vi "PenaltyAttackerSkill.vi"(8 "error in (no error)":errorcluster, 9 "Game":refnum<class "Game.lvclass">, 10 "Robot":refnum<class "Robot.lvclass">, 11 "PenaltyAttackerSkill in":refnum<class "PenaltyAttackerSkill.lvclass">) -> (0 "error out":errorcluster, 2 "Robot out":refnum<class "Robot.lvclass">, 3 "PenaltyAttackerSkill out":refnum<class "PenaltyAttackerSkill.lvclass">)   [LabVIEW 2018, in "PenaltyAttackerSkill.lvclass"]
uses:
  PenaltyAttackerSkill.lvclass
  Robot_class/Robot.lvclass
  C:/Users/yugon/Desktop/SSL_AI/SSL_AI/Object_class/Object.lvclass
  Game_class/Game.lvclass
  Utilities_class/Utilities.lvclass
  Game_class/Game.lvclass/Game.ctl
  Parameters_class/Parameters.lvclass/Parameters.ctl
  Team_class/Team.lvclass/Team.ctl
  Referee_class/Referee.lvclass/Referee.ctl
  Object_class/Object.lvclass/Object.ctl
  Robot_class/Robot.lvclass/Robot.ctl
  Team_class/Read RobotRef.vi
  Game_class/Read Parameters.lvclass.vi
  Parameters_class/Read KickForce.vi
  Object_class/Read x.vi
  Object_class/Read y.vi
  Game_class/Read FieldRef.vi
  Game_class/Read BallRef.vi
  Game_class/Read Referee.vi
  Game_class/Read AllyRef.vi
  Game_class/Read EnemyRef.vi
  Parameters_class/Read AttakingOurselves.vi
  Referee_class/Read enemy_goalie_id.vi
  Referee_class/Read our_goalie_id.vi
  Robot_class/Write dest_orientation.vi
  Robot_class/Write dest_x.vi
  Robot_class/Write dest_y.vi
  Robot_class/Write kick_x.vi
  Enemy_class/Enemy.lvclass
  C:/Users/yugon/Desktop/SSL_AI/SSL_AI/Team_class/Team.lvclass
  Ally_class/Ally.lvclass
  Ball_class/Ball.lvclass
  Referee_class/Referee.lvclass
  Parameters_class/Parameters.lvclass
  Field_class/Field.lvclass
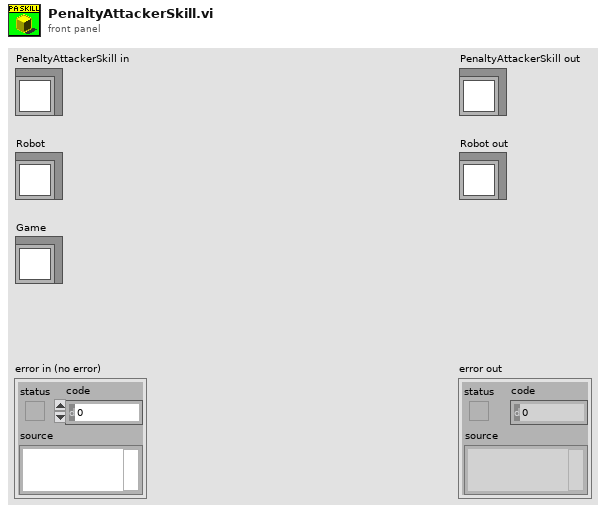
[diagram p1: front panel]
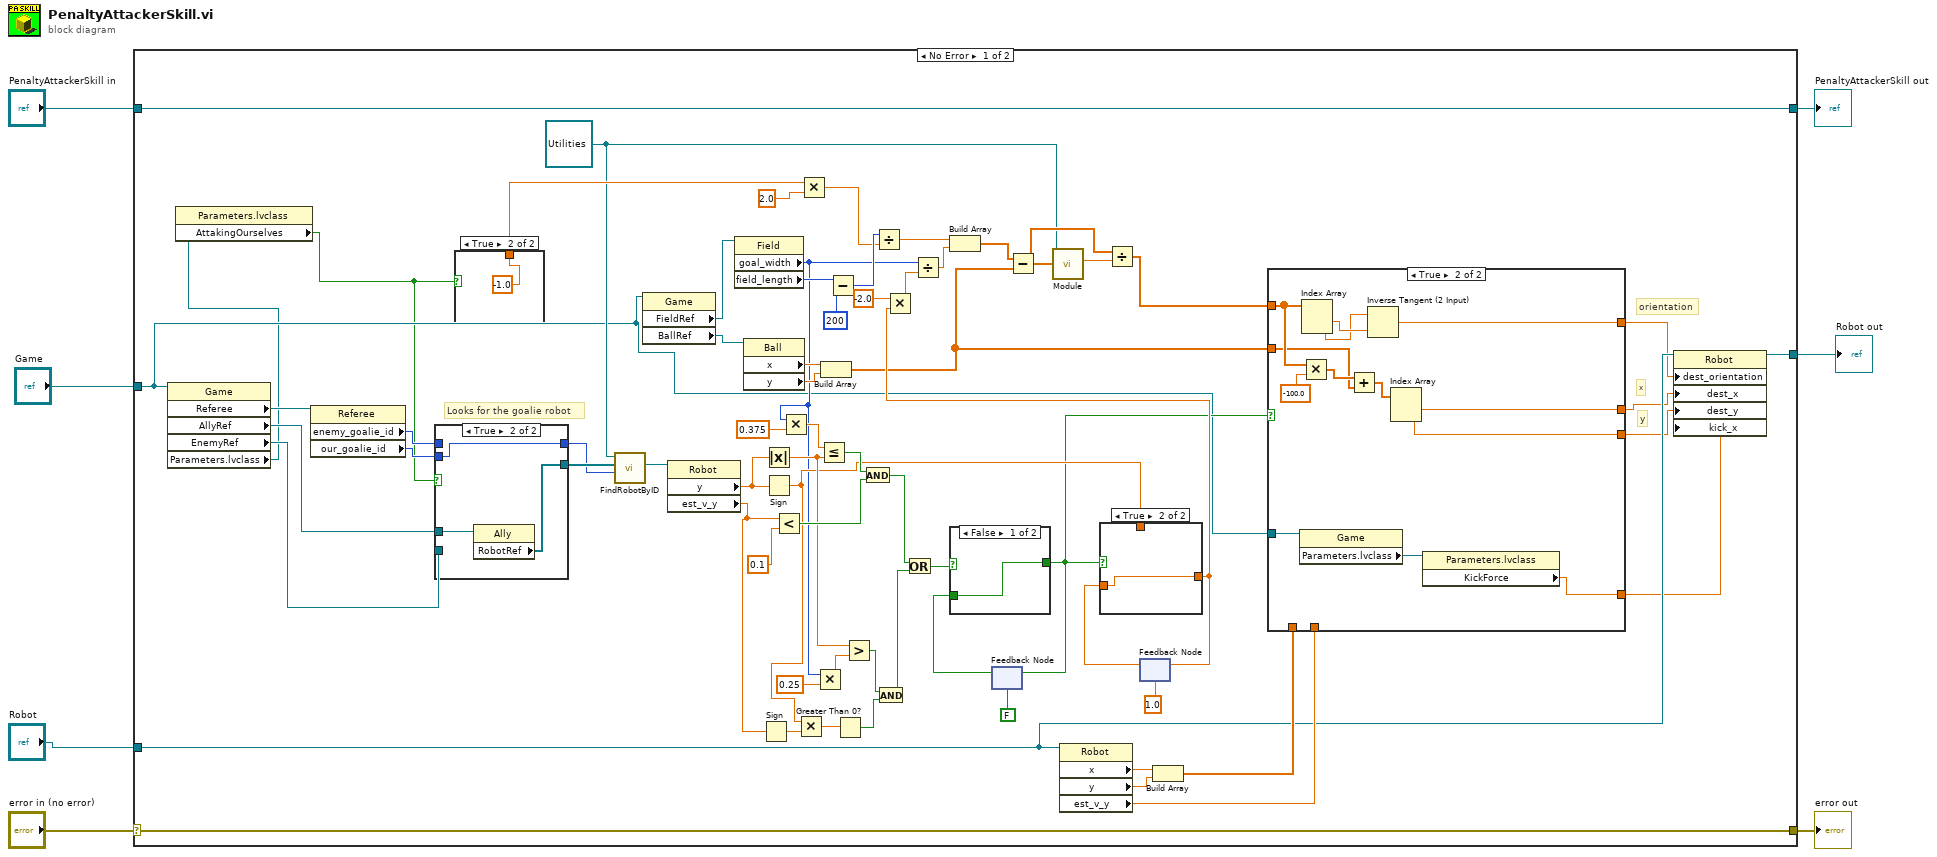
[diagram p0: block diagram]
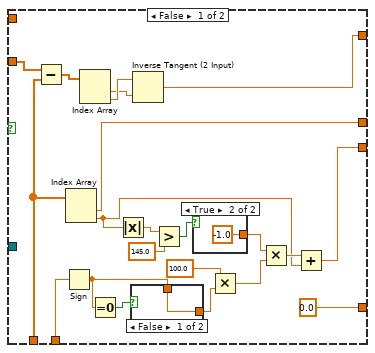
[diagram p2: hidden frame]
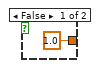
[diagram p3: hidden frame]
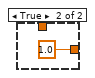
[diagram p4: hidden frame]
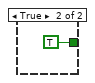
[diagram p6: hidden frame]
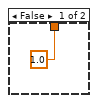
[diagram p7: hidden frame]
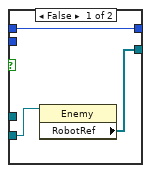
[diagram p8: hidden frame]
diagram:
  n1 = case shown="No Error" "error in (no error)" {
    selector: "error in (no error)" -> [w74 w128]
    tunnel: [w74 w128] -> w6
    tunnel: [w75 w127] -> w4
    tunnel: "PenaltyAttackerSkill in" -> [w75 w127]
    tunnel: "Game" -> [w10 _]
    tunnel: "Robot" -> [w17 w126]
    tunnel: [w13 w126] -> w1
    frame No Error {
      w12 = refnum<class "Utilities.lvclass"> refnum ("Utilities in")
      # "y"
      # "x"
      # "orientation"
      # "Looks for the goalie robot"
      n2 = property class="Game"(reference=w10) -> ("Referee"=w73:refnum<class "Referee.lvclass">, "AllyRef"=w72:refnum<class "Ally.lvclass">, "EnemyRef"=w71:refnum<class "Enemy.lvclass">, "Parameters.lvclass"=w9:refnum<class "Parameters.lvclass">)  [unwired: 1 in, 2 out]
      n3 = property class="Parameters.lvclass"(reference=w9) -> ("AttakingOurselves"=w8:bool)  [unwired: 1 in, 2 out]
      n4 = property class="Referee"(reference=w73) -> ("enemy_goalie_id"=w70:i32, "our_goalie_id"=w69:i32)  [unwired: 1 in, 2 out]
      n5 = case shown="True" w8 {
        tunnel: w72 -> [_ w125]
        tunnel: w71 -> [w122 _]
        tunnel: w70 -> [w120 _]
        tunnel: w69 -> [_ w123]
        tunnel: [w121 w124] -> w68
        tunnel: [w120 w123] -> w67
        frame False {
          n6 = property class="Enemy"(reference=w122) -> ("RobotRef"=w121:refnum<class "Robot.lvclass">[])  [unwired: 1 in, 2 out]
        }
        frame True {
          n7 = property class="Ally"(reference=w125) -> ("RobotRef"=w124:refnum<class "Robot.lvclass">[])  [unwired: 1 in, 2 out]
        }
      }
      n8 = case shown="True" w8 {
        tunnel: [1.0 -1.0] -> w39
        frame False {
        }
        frame True {
        }
      }
      n9 = call-dynamic "FindRobotByID.vi"("id"=w67, "RobotRef"=w68, "Utilities in"=w12) -> ("Robot"=w66:refnum<class "Robot.lvclass">)  [unwired: 5 in, 3 out]
      n10 = property class="Game"(reference=w10) -> ("FieldRef"=w65:refnum<class "Field.lvclass">, "BallRef"=w64:refnum<class "Ball.lvclass">)  [unwired: 1 in, 2 out]
      n11 = property class="Robot"(reference=w66) -> ("y"=w60:dbl, "est_v_y"=w52:dbl)  [unwired: 1 in, 2 out]
      n12 = property class="Field"(reference=w65) -> ("goal_width"=w31:i32, "field_length"=w37:i32)  [unwired: 1 in, 2 out]
      n13 = property class="Ball"(reference=w64) -> ("x"=w63:dbl, "y"=w62:dbl)  [unwired: 1 in, 2 out]
      n14 = Sign(1:w52) -> (0:w51:dbl)
      n15 = Absolute Value(x=w60) -> (abs(x)=w53:dbl)
      n16 = Sign(1:w60) -> (0:w42:dbl)
      n17 = Less?(x=w52, y=0.1) -> (x < y?=w56:bool)
      n18 = Multiply(x=w31, y=0.375) -> (x*y=w59:dbl)
      n19 = Multiply(x=w42, y=w51) -> (x*y=w50:dbl)
      n20 = Multiply(x=w39, y=2.0) -> (x*y=w34:dbl)
      n21 = Multiply(x=w31, y=0.25) -> (x*y=w54:dbl)
      n22 = Less Or Equal?(x=w59, y=w53) -> (x <= y?=w57:bool)
      n23 = Build Array(w63, w62) -> (w22:dbl[])
      n24 = Subtract(x=w37, y=200) -> (x-y=w35:i32)
      n25 = Greater Than 0?(x=w50) -> (x > 0?=w48:bool)
      n26 = Greater?(x=w53, y=w54) -> (0:w49:bool)
      n27 = And(x=w57, y=w56) -> (x .and. y?=w47:bool)
      n28 = Divide(x=w35, y=w34) -> (x/y=w33:dbl)
      n29 = And(x=w49, y=w48) -> (x .and. y?=w46:bool)
      n30 = Or(x=w47, y=w46) -> (x .or. y?=w45:bool)
      n31 = feedback #1(FALSE) -> (w44:bool)
      n32 = case shown="False" w45 {
        tunnel: [w116 TRUE] -> w24
        tunnel: w44 -> [w116 _]
        frame False {
        }
        frame True {
        }
      }
      n33 = feedback-in #1(w24) -> ()
      n34 = property class="Robot"(reference=w17) -> ("x"=w21:dbl, "y"=w20:dbl, "est_v_y"=w18:dbl)  [unwired: 1 in, 2 out]
      n35 = feedback #2(1.0) -> (w41:dbl)
      n36 = case shown="True" w24 {
        tunnel: w42 -> [w114 _]
        tunnel: [w114 w115] -> w29
        tunnel: w41 -> [_ w115]
        frame False {
        }
        frame True {
        }
      }
      n37 = Multiply(x=-2.0, y=w29) -> (x*y=w30:dbl)
      n38 = Divide(x=w31, y=w30) -> (x/y=w32:dbl)
      n39 = Build Array(w33, w32) -> (w27:dbl[])
      n40 = Subtract(x=w27, y=w22) -> (x-y=w25:dbl[])
      n41 = call-dynamic "Module.vi"("2D vector"=w25, "Utilities in"=w12) -> ("Modulo"=w26:dbl)  [unwired: 7 in, 2 out]
      n42 = Divide(x=w25, y=w26) -> (x/y=w23:dbl[])
      n43 = feedback-in #2(w29) -> ()
      n44 = Build Array(w21, w20) -> (w19:dbl[])
      n45 = case shown="True" w24 {
        tunnel: w23 -> [_ w111]
        tunnel: w22 -> [w96 w108]
        tunnel: w19 -> [w95 _]
        tunnel: [w79 w106] -> w15
        tunnel: [w77 w105] -> w14
        tunnel: [w91 w104] -> w16
        tunnel: w18 -> [w88 _]
        tunnel: [0.0 ("x") w101] -> w11
        tunnel: w10 -> [_ w103]
        frame False {
          n46 = Subtract(x=w96, y=w95) -> (x-y=w94:dbl[])
          n47 = Sign(1:w88) -> (0:w86:dbl)
          n48 = Index Array(array=w95) -> (element #1=w79:dbl, element #2=w78:dbl)  [unwired: 2 in]
          n49 = Index Array(array=w94) -> (element #1=w92:dbl, element #2=w93:dbl)  [unwired: 2 in]
          n50 = Equal To 0?(x=w86) -> (x = 0?=w87:bool)
          n51 = Absolute Value(x=w78) -> (abs(x)=w90:dbl)
          n52 = case shown="False" w87 {
            tunnel: [w99 1.0 ("y")] -> w85
            tunnel: w86 -> [w99 _]
            frame False {
            }
            frame True {
            }
          }
          n53 = Inverse Tangent (2 Input)(1:w92, 2:w93) -> (0:w91:dbl)
          n54 = Greater?(x=w90, y=145.0) -> (0:w83:bool)
          n55 = case shown="True" w83 {
            tunnel: [1.0 ("x") -1.0 ("x")] -> w82
            frame False {
            }
            frame True {
            }
          }
          n56 = Multiply(x=100.0, y=w85) -> (x*y=w81:dbl)
          n57 = Multiply(x=w82, y=w81) -> (x*y=w80:dbl)
          n58 = Add(x=w80, y=w78) -> (x+y=w77:dbl)
        }
        frame True {
          n59 = property class="Game"(reference=w103) -> ("Parameters.lvclass"=w102:refnum<class "Parameters.lvclass">)  [unwired: 1 in, 2 out]
          n60 = Multiply(x=w111, y=-100.0) -> (x*y=w109:dbl[])
          n61 = Index Array(array=w111) -> (element #1=w113:dbl, element #2=w112:dbl)  [unwired: 2 in]
          n62 = Add(x=w109, y=w108) -> (x+y=w107:dbl[])
          n63 = Inverse Tangent (2 Input)(1:w113, 2:w112) -> (0:w104:dbl)
          n64 = Index Array(array=w107) -> (element #1=w106:dbl, element #2=w105:dbl)  [unwired: 2 in]
          n65 = property class="Parameters.lvclass"(reference=w102) -> ("KickForce"=w101:dbl)  [unwired: 1 in, 2 out]
        }
      }
      n66 = property class="Robot"(reference=w17, "dest_orientation"=w16, "dest_x"=w15, "dest_y"=w14, "kick_x"=w11) -> (reference out=w13:refnum<class "Robot.lvclass">)  [unwired: 1 in, 1 out]
    }
    frame Error {
    }
  }
  "error out" <- w6
  "PenaltyAttackerSkill out" <- w4
  "Robot out" <- w1
